vi "Manual-Automatic Control.vi"() -> ()   [LabVIEW 2023]
doc: "This example uses the PID Advanced VI to switch between manual and automatic control. This VI also demonstrate how to use the beta parameter, also known as Setpoint Weighting. Changes in beta will reduce the setpoint change without altering the disturbance rejection."
uses:
  <vilib>/addons/control/pid/pid.llb/PID Structure.ctl
  <vilib>/addons/control/pid/pid.llb/PID Time Unit.ctl
  <vilib>/addons/control/pid/pid.llb/PID Gain Unit.ctl
  <vilib>/addons/control/pid/pid.llb/PID Structure Conversion (DBL).vi
  <vilib>/addons/control/pid/pid.llb/PID Advanced (DBL).vi
  <vilib>/addons/control/pid/NI_PID_pid.lvlib
panel:
  in  "PID Topology":T1 items=["Academic (Standard)", "Parallel", "Series"]
  in  "Proportional Unit":T2 items=["Gain (Kc)", "Band (PB)"]
  in  "Derivative Unit":T3 items=["min", "s"]
  in  "Integral Unit":T3 items=["min", "s"]
  in  "Derivative":dbl format="%#.3g"
  in  "Integral":dbl=0.008 format="%#.3g"
  in  "Proportional":dbl=5.0 format="%.3f"
  in  "Tab Control":enum32{"Instructions", "Charts"}(tab)
  out "Process Variable and Setpoint":cluster{"initial PV":dbl, "SP1:":dbl}(graph)={"initial PV"=59.99989543135817, "SP1:"=60.0}
  out "Controller Output":dbl(graph)=14.702188610163798
  in  "Fixed Load":dbl=40.0
  in  "Plant Load Profile":bool=TRUE
  out "PID Topology Equation":u16(ring) items=["PID Academic", "PID Parallel", "PID Series"]
  out "Plant Load (%)":u8(slide)=90 scale=0.0..100.0
  in  "Setpoint Profile":bool=TRUE
  in  "Auto?":bool=TRUE
  in  "SP:":dbl(slide)=60.0 scale=0.0..100.0
  in  "MV:":dbl(slide)=14.702188610163798 scale=-100.0..100.0 scale format="%#.3p"
  out "PV:":dbl(slide)=59.99989543135817 scale=0.0..100.0
  in  "Setpoint Weighting\n(Beta)":dbl(slide)=1.0 scale=0.0..1.0
  in  "Stop":bool
  # "Overview: Uses the PID Advanced VI to switch between manual and automatic control. This VI also demonstrates how to use Setpoint Weighting, or beta. Changes in beta reduce the setpoint change without altering the disturbance rejection.\nInstructions:\n1. Run the VI. Verify that there is a load disturbance, and then a setpoint change every 2 seconds, demonstrating the controller behavior under these conditions.\n2. Reduce the Setpoint Weighting (Beta) value to 0.2. Now, any setpoint change will not cause  the output response to overshoot, and it will keep the disturbance response with the same performance.\n3. Increase the Proportional gain to 10 and see how the disturbance is altered without setpoint changes.\n4. Make the controller Manual and move the slide of the Manipulated Variable (MV). Then, switch back to Automatic and verify how the controller tracks  the setpoint again.\n5. Change the gains of the controller to improve the controller performance. You can select the PID topology you are familiar with for tuning, and you can choose the parameter units.\n6. Click Stop to stop the VI."
  # "Automatic"
  # "Manual"
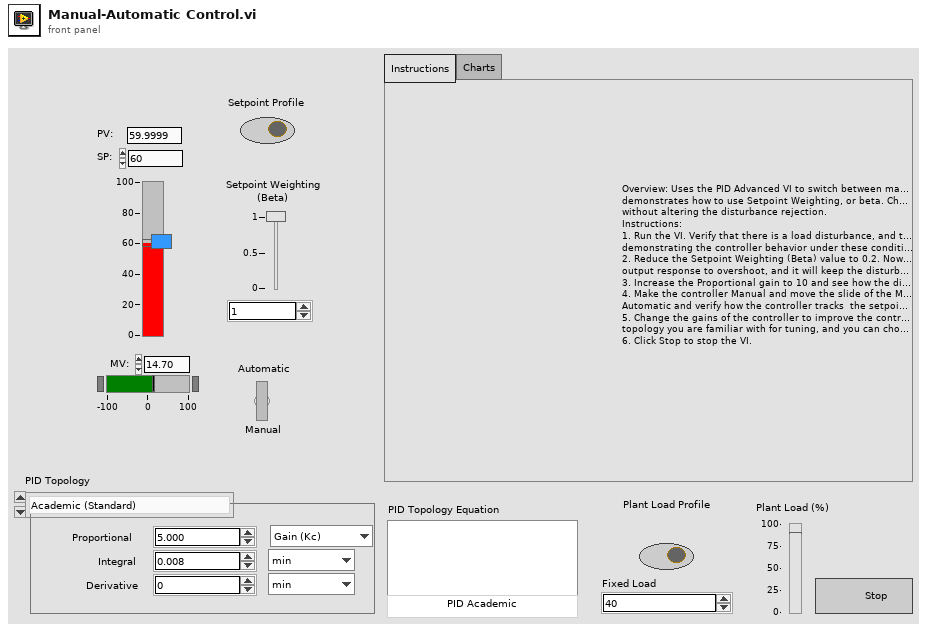
[diagram p1: front panel]
types:
  T1 = typedef "NI_PID_pid.lvlib/PID Structure.ctl" = u16
  T2 = typedef "NI_PID_pid.lvlib/PID Gain Unit.ctl" = u16
  T3 = typedef "NI_PID_pid.lvlib/PID Time Unit.ctl" = u16
  T4 = cluster{"static gain":dbl, "lag (min)":dbl, "dead cycles":dbl, "load %":dbl, "deadband":dbl, "noise level %":dbl, "initial PV":dbl, "noise level % 2":dbl}
  T5 = cluster{"proportional gain (Kc)":dbl, "integral time (Ti, min)":dbl, "derivative time (Td, min)":dbl}
  T6 = cluster{"Initial Process Variable (%)":dbl, "setpoint":dbl}
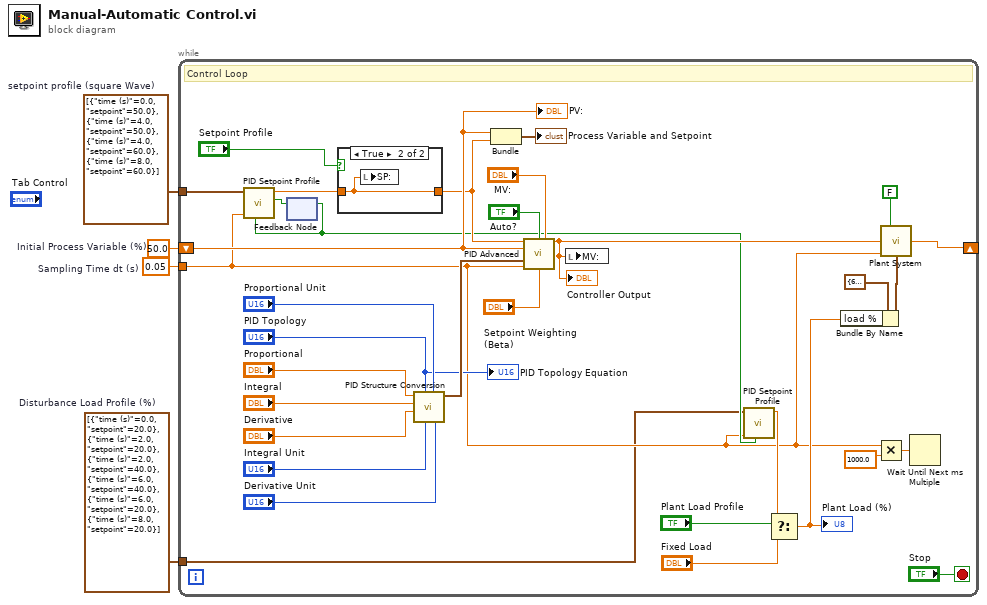
[diagram p0: block diagram]
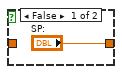
[diagram p2: hidden frame]
diagram:
  w1 = cluster{"time (s)":dbl, "setpoint":dbl}[] [{"time (s)"=0.0, "setpoint"=20.0}, {"time (s)"=2.0, "setpoint"=20.0}, {"time (s)"=2.0, "setpoint"=40.0}, {"time (s)"=6.0, "setpoint"=40.0}, {"time (s)"=6.0, "setpoint"=20.0}, {"time (s)"=8.0, "setpoint"=20.0}]  # Disturbance Load Profile (%)
  w2 = 0.05  # Sampling Time dt (s)
  w4 = 50.0  # Initial Process Variable (%)
  w3 = cluster{"time (s)":dbl, "setpoint":dbl}[] [{"time (s)"=0.0, "setpoint"=50.0}, {"time (s)"=4.0, "setpoint"=50.0}, {"time (s)"=4.0, "setpoint"=60.0}, {"time (s)"=8.0, "setpoint"=60.0}]  # setpoint profile (square Wave)
  n1 = while {
    shift-left: w4 -> [w25]
    shift-right: [w8] -> _
    tunnel: w3 -> [w21]
    tunnel: w2 -> [w6]
    tunnel: w1 -> [w5]
    stop <- "Stop" stop-if-true
    # "Control Loop"
    n2 = feedback #1() -> (w17:bool)  [unwired: 1 in]
    n3 = call <vilib>:"PID Setpoint Profile.vi"("reinitialize? (F)"=w17, "dt (s)"=w6, "setpoint profile"=w21) -> ("profile complete?"=w20:bool, "setpoint"=w18:dbl)  [unwired: 3 in, 2 out]
    n4 = feedback-in #1(w20) -> ()
    n5 = case shown="True" "Setpoint Profile" {
      tunnel: ["SP:" w39] -> w24
      tunnel: w18 -> [_ w39]
      frame False {
      }
      frame True {
        n6 = local write "SP:"(w39) -> ()
      }
    }
    n7 = call-poly <vilib>:"PID Structure Conversion.vi"("derivative unit"="Derivative Unit", "proportional unit"="Proportional Unit", "integral unit"="Integral Unit", "PID structure"="PID Topology", "derivative"="Derivative", "integral"="Integral", "proportional"="Proportional") -> ("PID gains"=w31:T5)  [unwired: 4 in]
    n8 = Bundle("Initial Process Variable (%)"=w25, "setpoint"=w24) -> (→"Process Variable and Setpoint":T6)  [unwired: 1 in]
    n9 = call-poly <vilib>:"PID Advanced.vi"("setpoint"=w24, "auto? (T)"="Auto?", "manual control"="MV:", "process variable"=w25, "PID gains"=w31, "dt (s)"=w6, "beta"="Setpoint Weighting\n(Beta)") -> ("output"=w22:dbl)  [unwired: 7 in, 1 out]
    "Controller Output" <- w22
    n10 = local write "MV:"(w22) -> ()
    n11 = call <vilib>:"PID Setpoint Profile.vi"("reinitialize? (F)"=w17, "dt (s)"=w6, "setpoint profile"=w5) -> ("setpoint"=w16:dbl)  [unwired: 3 in, 3 out]
    n12 = Select(t=w16, s="Plant Load Profile", f="Fixed Load") -> (s? t:f=w9:dbl)
    "Plant Load (%)" <- w9
    n13 = Bundle By Name(cluster=T4 {"static gain"=6.0, "lag (min)"=6.0, "dead cycles"=0.0, "load %"=40.0, "deadband"=0.0, "noise level %"=0.0, "initial PV"=50.0, "noise level % 2"=0.0} ("process parameters"), "load %"=w9) -> (w11:T4)
    n14 = Multiply(x=w6, y=1000.0) -> (x*y=w7:dbl)
    n15 = call "Plant System.vi"("Integrator ?"=FALSE, "Plant Input"=w22, "dt (s)"=w6, "process parameters"=w11) -> ("Plant Output"=w8:dbl)  [unwired: 11 in]
    n16 = Wait Until Next ms Multiple(millisecond multiple=w7) -> ()  [unwired: 1 out]
    "PV:" <- w25
    "PID Topology Equation" <- "PID Topology"
  }
